vi "Sollwert AutiLIN MFC Abfragen.vi"   [LabVIEW 2020, in "Linearisierung v2.lvlib" / "Gasteiler.lvlib" / "HovaCAL_Interface.lvlib" / "Kommunikation.lvlib"]
uses:
  Kommunikation.lvlib
  Aktion FGV HovaCAL Interface Autolin.ctl
  Aktion FGV Rohmesswerte sammeln.ctl
  Linearisierung v2.lvlib
  Helper/Helper.lvlib
types:
  T1 = typedef "Linearisierung v2.lvlib/Gasteiler.lvlib/HovaCAL_Interface.lvlib/Kommunikation.lvlib/Aktion FGV HovaCAL Interface Autolin.ctl" = enum16{"lesen", "schreiben", "MFC Komponente fix setzen", "init"}
  T2 = typedef "Linearisierung v2.lvlib/Aktion FGV Rohmesswerte sammeln.ctl" = enum16{"lesen", "schreiben", "löschen", "Sollwert HovaCal"}
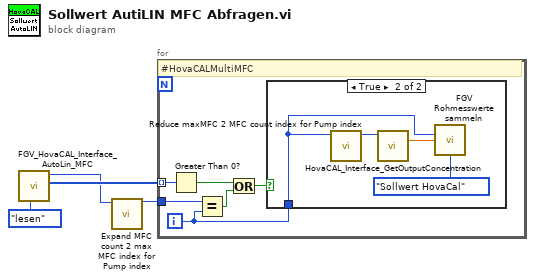
[diagram p0: block diagram]
diagram:
  n1 = call "FGV_HovaCAL_Interface_AutoLin_MFC.vi"("Aktion"=Aktion_FGV_HovaCAL_Interface_Autolin."lesen") -> ("MFV Komponente fix out"=w3:u16[], "AutoLin MFC out"=w1:u16)  [unwired: 7 in, 2 out]
  n2 = call "Expand MFC count 2 max MFC index for Pump index.vi"("AutoLin MFC"=w1) -> ("MFC idx"=w2:i32)  [unwired: 8 in, 2 out]
  n3 = for {
    tunnel: w3 -> [w10] mode=indexing
    tunnel: w2 -> [w5]
    i -> [w7]
    # "#HovaCALMultiMFC"
    n4 = Greater Than 0?(x=w10) -> (x > 0?=w9:bool)
    n5 = Equal?(x=w5, y=w7) -> (x = y?=w6:bool)
    n6 = Or(x=w9, y=w6) -> (x .or. y?=w8:bool)
    n7 = case shown="True" w8 {
      tunnel: w7 -> [_ w11]
      frame False {
      }
      frame True {
        n8 = call "Reduce maxMFC 2 MFC count index for Pump index.vi"("MFC idx"=w11) -> ("AutoLin MFC"=w13:i32)  [unwired: 8 in, 2 out]
        n9 = call "HovaCAL_Interface_GetOutputConcentration.vi"("AutoLin MFC Index"=w13) -> ("Konzentration"=w12:dbl)  [unwired: 8 in, 2 out]
        n10 = call "FGV Rohmesswerte sammeln.vi"("MFC in"=w11, "Sollwert"=w12, "Aktion"=Aktion_FGV_Rohmesswerte_sammeln."Sollwert HovaCal") -> ()  [unwired: 9 in, 4 out]
      }
    }
  }
